vi "Leitura_de_TXT.vi"() -> ()   [LabVIEW 2014]
uses:
  leitura de dados txt control.ctl
  <vilib>/Utility/file.llb/Read From Spreadsheet File (string).vi
  <vilib>/gmath/NI_Gmath.lvlib
panel:
  out "XY Graph":T1(graph)
  out "GammaInterval":dbl[](array[numeric])
  out "Interpolated":dbl[][](array[numeric])
  out "NeedInterpolation?":bool
  out "Collumns":i32
  out "Rows":i32
  out "Illuminant Tabel":string[][](array[string])
  out "Selected illuminant index":dbl
  in  "ComboBox Illuminant":T2
  # "Selecione o iluminante que deseja utilizar."
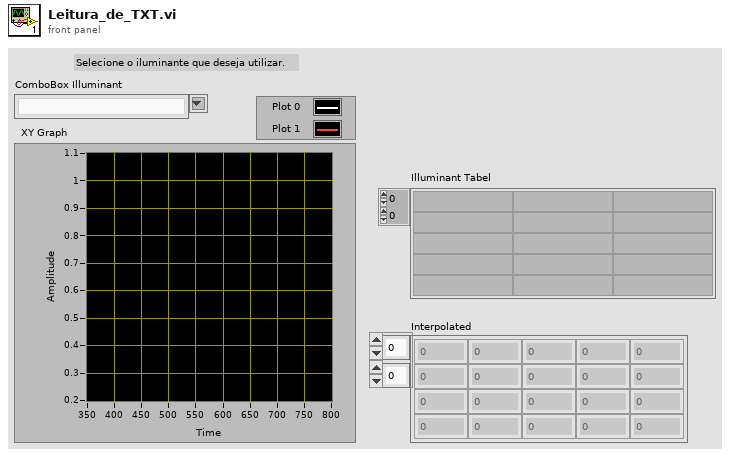
[diagram p1: front panel]
types:
  T1 = cluster{"GammaInterval":dbl[], "Interpolated":dbl[]}[]
  T2 = typedef "leitura de dados txt control.ctl" = string
  T3 = typedef "Control 1" = string
  T4 = cluster{"GammaInterval":dbl[], "Interpolated":dbl[]}
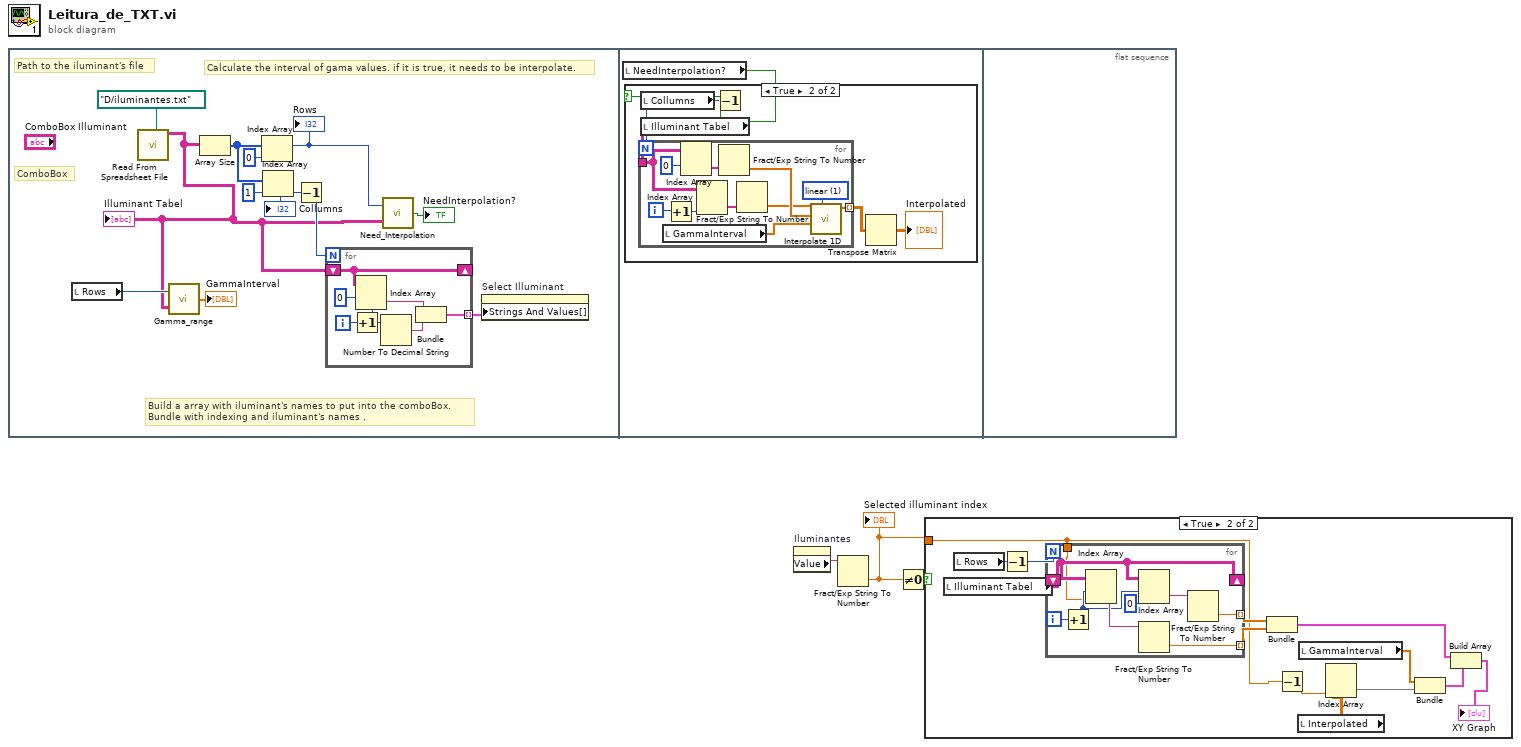
[diagram p0: block diagram]
diagram:
  n1 = flat-sequence {
    frame #0 {
      # "Calculate the interval of gama values. if it is true, it needs to be interpolate."
      # "Path to the iluminant's file"
      # "ComboBox"
      # "Build a array with iluminant's names to put into the comboBox.\nBundle with indexing and iluminant's names ."
      n2 = local read "Rows"() -> (w8:i32)
      n3 = call-poly <vilib>:"Read From Spreadsheet File.vi"("file path (dialog if empty)"=path "D:/iluminantes.txt") -> ("all rows"=w4:string[][])  [unwired: 6 in, 4 out]
      "Illuminant Tabel" <- w4
      n4 = call "Gamma_range.vi"("Illuminant Table"=w4, "NumberOfRows"=w8) -> ("GammaInterval"=→"GammaInterval":dbl[])
      n5 = Array Size(array=w4) -> (size(s)=w11:i32[])
      n6 = Index Array(array=w11, index=0) -> (element=w5:i32)
      "Rows" <- w5
      n7 = Index Array(array=w11, index=1) -> (element=w13:i32)
      "Collumns" <- w13
      n8 = Decrement(x=w13) -> (x-1=w14:i32)
      n9 = for {
        N: w14 -> [_]
        shift-right: [w20] -> _
        shift-left: w4 -> [w20]
        tunnel: [w16] -> w15 mode=indexing
        i -> [w22]
        n10 = Increment(x=w22) -> (x+1=w19:i32)
        n11 = Index Array(array=w20, index (row)=0, index (col)=w19) -> (element=w17:string)
        n12 = Number To Decimal String(number=w19) -> (decimal integer string=w18:string)  [unwired: 1 in]
        n13 = Bundle("String"=w17, w18) -> (w16:cluster{"String":string, string})  [unwired: 1 in]
      }
      n14 = call "Need_Interpolation.vi"("Matrix with txt"=w4, "Number of Rows"=w5) -> ("isNotFive?"=→"NeedInterpolation?":bool)
      n15 = property on="Select Illuminant" class="CmbBox (strict)"("Strings And Values[]"=w15) -> ()  [unwired: 2 in, 2 out]
    }
    frame #1 {
      n16 = local read "NeedInterpolation?"() -> (w23:bool)
      n17 = case shown="True" w23 {
        frame False {
        }
        frame True {
          n18 = local read "Collumns"() -> (w25:i32)
          n19 = local read "Illuminant Tabel"() -> (w28:string[][])
          n20 = Decrement(x=w25) -> (x-1=w24:i32)
          n21 = for {
            N: w24 -> [_]
            tunnel: w28 -> [w36]
            tunnel: [w33] -> w27 mode=indexing
            i -> [w32]
            w29 = 1 items=["nearest", "linear", "spline", "cubic Hermite", "Lagrange"] ("method")
            n22 = local read "GammaInterval"() -> (w30:dbl[])
            n23 = Increment(x=w32) -> (x+1=w31:i32)
            n24 = Index Array(array=w36, index (col)=0 ("disabled index (col)")) -> (element=w38:string[])  [unwired: 1 in]
            n25 = Index Array(array=w36, index (col)=w31) -> (element=w35:string[])  [unwired: 1 in]
            n26 = Fract/Exp String To Number(string=w38) -> (number=w37:dbl[])  [unwired: 3 in, 1 out]
            n27 = Fract/Exp String To Number(string=w35) -> (number=w34:dbl[])  [unwired: 3 in, 1 out]
            n28 = call <vilib>:"Interpolate 1D.vi"("method"=w29, "xi"=w30, "X"=w37, "Y"=w34) -> ("yi"=w33:dbl[])  [unwired: 5 in, 2 out]
          }
          n29 = Transpose Matrix(1:w27) -> (0:→"Interpolated":dbl[][])
        }
      }
    }
    frame #2 {
    }
  }
  n30 = property on="Iluminantes" class="CmbBox (strict)"() -> ("Value"=w3:T3)  [unwired: 2 in, 2 out]
  n31 = Fract/Exp String To Number(string=w3) -> (number=w1:dbl)  [unwired: 3 in, 1 out]
  "Selected illuminant index" <- w1
  n32 = Not Equal To 0?(x=w1) -> (x != 0?=w2:bool)
  n33 = case shown="True" w2 {
    tunnel: w1 -> [_ w41]
    frame False {
    }
    frame True {
      n34 = local read "Illuminant Tabel"() -> (w50:string[][])
      n35 = local read "Rows"() -> (w51:i32)
      n36 = Decrement(x=w51) -> (x-1=w52:i32)
      n37 = for {
        N: w52 -> [_]
        shift-right: [w60] -> _
        shift-left: w50 -> [w60]
        tunnel: w41 -> [w53]
        tunnel: [w55] -> w49 mode=indexing
        tunnel: [w54] -> w48 mode=indexing
        i -> [w61]
        n38 = Increment(x=w61) -> (x+1=w56:i32)
        n39 = Index Array(array=w60, index (row)=w56, index (col)=w53) -> (element=w57:string)
        n40 = Index Array(array=w60, index (row)=w56, index (col)=0 ("disabled index (col)")) -> (element=w58:string)
        n41 = Fract/Exp String To Number(string=w57) -> (number=w55:dbl)  [unwired: 3 in, 1 out]
        n42 = Fract/Exp String To Number(string=w58) -> (number=w54:dbl)  [unwired: 3 in, 1 out]
      }
      n43 = Bundle(w48, w49) -> (w42:cluster{dbl[], dbl[]})  [unwired: 1 in]
      n44 = Decrement(x=w41) -> (x-1=w40:dbl)
      n45 = local read "Interpolated"() -> (w43:dbl[][])
      n46 = local read "GammaInterval"() -> (w44:dbl[])
      n47 = Index Array(array=w43, index (col)=w40) -> (element=w45:dbl[])  [unwired: 1 in]
      n48 = Bundle("GammaInterval"=w44, "Interpolated"=w45) -> (w46:T4)  [unwired: 1 in]
      n49 = Build Array(w42, w46) -> (→"XY Graph":T1)
    }
  }
